vi "WildDrive_v5.0.vi"(6 "Selected_Driver":i32, 8 "Super Turn":bool, 9 "Legal_Drivers":string[](array[string])=["Ethan", "Adam", "Amelia"], 10 "Turn Joystick":dbl, 11 "Speed Joystick":dbl=-0.0) -> (0 "Right Side Power":dbl, 3 "Left Side Power":dbl)   [LabVIEW 2019]
doc: "This VI is designed for use with a butterfly drive, although it can be adapted for use with other differential drive systems. Essentially, this algorithm provides a smooth transition between two different turning modes. At lower speeds the robot will pivot about its center axis while at higher speeds the robot will perform an arc turn. Smooth transitions from deadbands and additional limits on the max pivot turn speed are supported. Toggle \"Turn Behavior\" to steer like car or steer like a traditional FRC robot when driving backwards. Do NOT enter \"Debug Mode\" while the robot is enabled. Do NOT leave \"Synce Driver Profile\" enabled when permenantly deployed to the robot (b/c certain GUI actions are not supported by he RoboRIO). Driver profiles are supported although selection (i.e. via the dashboard) is left to the user."
uses:
  <vilib>/Analysis/1siggen.llb/Ramp Pattern by Samples.vi
  <vilib>/Analysis/NI_AALBase.lvlib
panel:
  in  "Sync Driver Profile":bool
  out "Current_Driver":string
  in  "Feed Forward Coeff":dbl[](array[slide])=[0.05, 0.05, 0.05] min=0.0 max=0.2 scale=0.0..0.2
  in  "Mixing Coefficient":dbl[](array[slide])=[20.0, 20.0, 25.0] min=1.0 max=100.0 scale=1.0..100.0
  in  "Max Pivot Turn (super)":dbl[](array[slide])=[1.0, 1.0, 1.0] min=0.0 max=1.0 scale=0.0..1.0
  in  "Max Pivot Turn (normal)":dbl[](array[slide])=[0.8, 0.8, 0.5] min=0.0 max=1.0 scale=0.0..1.0
  in  "Tune Arc Turn":dbl[](array[slide])=[1.2, 1.2, 0.9] min=0.9 max=2.0 scale=0.9..2.0
  in  "Speed Joystick Deadband":dbl[](array[slide])=[0.05, 0.05, 0.05] min=0.0 max=1.0 scale=0.0..1.0
  in  "Turning Joystick Deadband":dbl[](array[slide])=[0.05, 0.1, 0.2] min=0.0 max=1.0 scale=0.0..1.0
  out "Mixing Function":cluster{"Y":dbl[], "X":dbl[]}(graph)={"Y"=[0.0, 0.010101010101010102, 0.020202020202020204, 0.030303030303030304, 0.04040404040404041, 0.05050505050505051, 0.06060606060606061, 0.07070707070707072, 0.08080808080808081, 0.09090909090909091, 0.10101010101010102, 0.11111111111111112, 0.12121212121212122, 0.13131313131313133, 0.14141414141414144, 0.15151515151515152, 0.16161616161616163, 0.17171717171717174, 0.18181818181818182, 0.19191919191919193, 0.20202020202020204, 0.21212121212121213, 0.22222222222222224, 0.23232323232323235, 0.24242424242424243, 0.25252525252525254, 0.26262626262626265, 0.27272727272727276, 0.2828282828282829, 0.29292929292929293, 0.30303030303030304, 0.31313131313131315, 0.32323232323232326, 0.33333333333333337, 0.3434343434343435, 0.3535353535353536, 0.36363636363636365, 0.37373737373737376, 0.38383838383838387, 0.393939393939394, 0.4040404040404041, 0.4141414141414142, 0.42424242424242425, 0.43434343434343436, 0.4444444444444445, 0.4545454545454546, 0.4646464646464647, 0.4747474747474748, 0.48484848484848486, 0.494949494949495, 0.5050505050505051, 0.5151515151515152, 0.5252525252525253, 0.5353535353535354, 0.5454545454545455, 0.5555555555555556, 0.5656565656565657, 0.5757575757575758, 0.5858585858585859, 0.595959595959596, 0.6060606060606061, 0.6161616161616162, 0.6262626262626263, 0.6363636363636365, 0.6464646464646465, 0.6565656565656566, 0.6666666666666667, 0.6767676767676768, 0.686868686868687, 0.696969696969697, 0.7070707070707072, 0.7171717171717172, 0.7272727272727273, 0.7373737373737375, 0.7474747474747475, 0.7575757575757577, 0.7676767676767677, 0.7777777777777778, 0.787878787878788, 0.797979797979798, 0.8080808080808082, 0.8181818181818182, 0.8282828282828284, 0.8383838383838385, 0.8484848484848485, 0.8585858585858587, 0.8686868686868687, 0.8787878787878789, 0.888888888888889, 0.8989898989898991, 0.9090909090909092, 0.9191919191919192, 0.9292929292929294, 0.9393939393939394, 0.9494949494949496, 0.9595959595959597, 0.9696969696969697, 0.9797979797979799, 0.98989898989899, 1.0], "X"=[1.0, 0.36603234127322715, 0.13532626064379283, 0.05052453015628186, 0.019045702193466962, 0.007247455040202033, 0.002783489278110511, 0.0010787801167675484, 0.00042183410694076207, 0.00016639639425326962, 6.620177984839095e-05, 2.6561398887587357e-05, 1.0745375115522577e-05, 4.382452248980866e-06, 1.8016694372108035e-06, 7.465077591438598e-07, 3.1169901107319554e-07, 1.3113557868070773e-07, 5.5581886768235786e-08, 2.373114697909272e-08, 1.0205242300096137e-08, 4.419721001217318e-09, 1.927446925622597e-09, 8.463234846310681e-10, 3.7411775176233565e-10, 1.6647573596881723e-10, 7.456210476755159e-11, 3.360972414714873e-11, 1.5245699808641053e-11, 6.958609969858144e-12, 3.195570695186819e-12, 1.4763326653758367e-12, 6.86103909791559e-13, 3.2072021853814684e-13, 1.5078403574264123e-13, 7.129180709244532e-14, 3.3895544142624165e-14, 1.6204238353260086e-14, 7.788659967873636e-15, 3.76366378038304e-15, 1.82826621688999e-15, 8.927212895741967e-16, 4.381352486286385e-16, 2.1611505485274178e-16, 1.0713113677174099e-16, 5.336668792886832e-17, 2.6712789155004126e-17, 1.3434882772756658e-17, 6.788690117455716e-18, 3.4462590553247523e-18, 1.7574890123257356e-18, 9.003130684840785e-19, 4.632599227711995e-19, 2.394201316530436e-19, 1.2427288424976475e-19, 6.478095947844572e-20, 3.391170633552417e-20, 1.782623487107148e-20, 9.409232908362009e-21, 4.986671552400837e-21, 2.6534262895136237e-21, 1.4174938853880581e-21, 7.602069865092925e-22, 4.0927762769197154e-22, 2.211867051717034e-22, 1.1998712710421777e-22, 6.53318623500068e-23, 3.570348880574086e-23, 1.958268982155976e-23, 1.0779318073480446e-23, 5.95455071339927e-24, 3.300861649468989e-24, 1.8361511142543956e-24, 1.0248841317144169e-24, 5.739963712987115e-25, 3.2254820658410615e-25, 1.8185053837023498e-25, 1.0286145857915951e-25, 5.837042071494194e-26, 3.3229149745670054e-26, 1.8976510791597504e-26, 1.0870986324891945e-26, 6.246862874883761e-27, 3.6006479544686514e-27, 2.0816633052912476e-27, 1.2070830701485794e-27, 7.020153679465042e-28, 4.094727808938361e-28, 2.3952938868546393e-28, 1.4051883268944269e-28, 8.266830677466088e-29, 4.877074216359946e-29, 2.8852452517622416e-29, 1.711577581520392e-29, 1.0180955963877349e-29, 6.0722055822989395e-30, 3.6312681754960745e-30, 2.1772701780581707e-30, 1.3088709946601708e-30, 7.888609052210118e-31]}
  in  "Debug Mode":bool
  in  "Debug Speed":dbl(slide) min=0.0 max=1.0 scale=0.0..1.0
  in  "Square Speed":bool=TRUE
  in  "Turn Behavior":bool=TRUE
  out "Left Side Power":cluster{"Y":dbl[], "X":dbl[]}(graph)={"Y"=[0.0, 0.010101010101010102, 0.020202020202020204, 0.030303030303030304, 0.04040404040404041, 0.05050505050505051, 0.06060606060606061, 0.07070707070707072, 0.08080808080808081, 0.09090909090909091, 0.10101010101010102, 0.11111111111111112, 0.12121212121212122, 0.13131313131313133, 0.14141414141414144, 0.15151515151515152, 0.16161616161616163, 0.17171717171717174, 0.18181818181818182, 0.19191919191919193, 0.20202020202020204, 0.21212121212121213, 0.22222222222222224, 0.23232323232323235, 0.24242424242424243, 0.25252525252525254, 0.26262626262626265, 0.27272727272727276, 0.2828282828282829, 0.29292929292929293, 0.30303030303030304, 0.31313131313131315, 0.32323232323232326, 0.33333333333333337, 0.3434343434343435, 0.3535353535353536, 0.36363636363636365, 0.37373737373737376, 0.38383838383838387, 0.393939393939394, 0.4040404040404041, 0.4141414141414142, 0.42424242424242425, 0.43434343434343436, 0.4444444444444445, 0.4545454545454546, 0.4646464646464647, 0.4747474747474748, 0.48484848484848486, 0.494949494949495, 0.5050505050505051, 0.5151515151515152, 0.5252525252525253, 0.5353535353535354, 0.5454545454545455, 0.5555555555555556, 0.5656565656565657, 0.5757575757575758, 0.5858585858585859, 0.595959595959596, 0.6060606060606061, 0.6161616161616162, 0.6262626262626263, 0.6363636363636365, 0.6464646464646465, 0.6565656565656566, 0.6666666666666667, 0.6767676767676768, 0.686868686868687, 0.696969696969697, 0.7070707070707072, 0.7171717171717172, 0.7272727272727273, 0.7373737373737375, 0.7474747474747475, 0.7575757575757577, 0.7676767676767677, 0.7777777777777778, 0.787878787878788, 0.797979797979798, 0.8080808080808082, 0.8181818181818182, 0.8282828282828284, 0.8383838383838385, 0.8484848484848485, 0.8585858585858587, 0.8686868686868687, 0.8787878787878789, 0.888888888888889, 0.8989898989898991, 0.9090909090909092, 0.9191919191919192, 0.9292929292929294, 0.9393939393939394, 0.9494949494949496, 0.9595959595959597, 0.9696969696969697, 0.9797979797979799, 0.98989898989899, 1.0], "X"=[0.0]}
  out "Right Side Power":cluster{"Y":dbl[], "X":dbl[]}(graph)={"Y"=[0.0, 0.010101010101010102, 0.020202020202020204, 0.030303030303030304, 0.04040404040404041, 0.05050505050505051, 0.06060606060606061, 0.07070707070707072, 0.08080808080808081, 0.09090909090909091, 0.10101010101010102, 0.11111111111111112, 0.12121212121212122, 0.13131313131313133, 0.14141414141414144, 0.15151515151515152, 0.16161616161616163, 0.17171717171717174, 0.18181818181818182, 0.19191919191919193, 0.20202020202020204, 0.21212121212121213, 0.22222222222222224, 0.23232323232323235, 0.24242424242424243, 0.25252525252525254, 0.26262626262626265, 0.27272727272727276, 0.2828282828282829, 0.29292929292929293, 0.30303030303030304, 0.31313131313131315, 0.32323232323232326, 0.33333333333333337, 0.3434343434343435, 0.3535353535353536, 0.36363636363636365, 0.37373737373737376, 0.38383838383838387, 0.393939393939394, 0.4040404040404041, 0.4141414141414142, 0.42424242424242425, 0.43434343434343436, 0.4444444444444445, 0.4545454545454546, 0.4646464646464647, 0.4747474747474748, 0.48484848484848486, 0.494949494949495, 0.5050505050505051, 0.5151515151515152, 0.5252525252525253, 0.5353535353535354, 0.5454545454545455, 0.5555555555555556, 0.5656565656565657, 0.5757575757575758, 0.5858585858585859, 0.595959595959596, 0.6060606060606061, 0.6161616161616162, 0.6262626262626263, 0.6363636363636365, 0.6464646464646465, 0.6565656565656566, 0.6666666666666667, 0.6767676767676768, 0.686868686868687, 0.696969696969697, 0.7070707070707072, 0.7171717171717172, 0.7272727272727273, 0.7373737373737375, 0.7474747474747475, 0.7575757575757577, 0.7676767676767677, 0.7777777777777778, 0.787878787878788, 0.797979797979798, 0.8080808080808082, 0.8181818181818182, 0.8282828282828284, 0.8383838383838385, 0.8484848484848485, 0.8585858585858587, 0.8686868686868687, 0.8787878787878789, 0.888888888888889, 0.8989898989898991, 0.9090909090909092, 0.9191919191919192, 0.9292929292929294, 0.9393939393939394, 0.9494949494949496, 0.9595959595959597, 0.9696969696969697, 0.9797979797979799, 0.98989898989899, 1.0], "X"=[0.0]}
  out "Speed Joystick Mapping":cluster{"Y":dbl[], "X":dbl[]}(graph)={"Y"=[0.0, 0.010101010101010102, 0.020202020202020204, 0.030303030303030304, 0.04040404040404041, 0.05050505050505051, 0.06060606060606061, 0.07070707070707072, 0.08080808080808081, 0.09090909090909091, 0.10101010101010102, 0.11111111111111112, 0.12121212121212122, 0.13131313131313133, 0.14141414141414144, 0.15151515151515152, 0.16161616161616163, 0.17171717171717174, 0.18181818181818182, 0.19191919191919193, 0.20202020202020204, 0.21212121212121213, 0.22222222222222224, 0.23232323232323235, 0.24242424242424243, 0.25252525252525254, 0.26262626262626265, 0.27272727272727276, 0.2828282828282829, 0.29292929292929293, 0.30303030303030304, 0.31313131313131315, 0.32323232323232326, 0.33333333333333337, 0.3434343434343435, 0.3535353535353536, 0.36363636363636365, 0.37373737373737376, 0.38383838383838387, 0.393939393939394, 0.4040404040404041, 0.4141414141414142, 0.42424242424242425, 0.43434343434343436, 0.4444444444444445, 0.4545454545454546, 0.4646464646464647, 0.4747474747474748, 0.48484848484848486, 0.494949494949495, 0.5050505050505051, 0.5151515151515152, 0.5252525252525253, 0.5353535353535354, 0.5454545454545455, 0.5555555555555556, 0.5656565656565657, 0.5757575757575758, 0.5858585858585859, 0.595959595959596, 0.6060606060606061, 0.6161616161616162, 0.6262626262626263, 0.6363636363636365, 0.6464646464646465, 0.6565656565656566, 0.6666666666666667, 0.6767676767676768, 0.686868686868687, 0.696969696969697, 0.7070707070707072, 0.7171717171717172, 0.7272727272727273, 0.7373737373737375, 0.7474747474747475, 0.7575757575757577, 0.7676767676767677, 0.7777777777777778, 0.787878787878788, 0.797979797979798, 0.8080808080808082, 0.8181818181818182, 0.8282828282828284, 0.8383838383838385, 0.8484848484848485, 0.8585858585858587, 0.8686868686868687, 0.8787878787878789, 0.888888888888889, 0.8989898989898991, 0.9090909090909092, 0.9191919191919192, 0.9292929292929294, 0.9393939393939394, 0.9494949494949496, 0.9595959595959597, 0.9696969696969697, 0.9797979797979799, 0.98989898989899, 1.0], "X"=[0.0]}
  out "Turn Joystick Mapping":cluster{"Y":dbl[], "X":dbl[]}(graph)={"Y"=[0.0, 0.010101010101010102, 0.020202020202020204, 0.030303030303030304, 0.04040404040404041, 0.05050505050505051, 0.06060606060606061, 0.07070707070707072, 0.08080808080808081, 0.09090909090909091, 0.10101010101010102, 0.11111111111111112, 0.12121212121212122, 0.13131313131313133, 0.14141414141414144, 0.15151515151515152, 0.16161616161616163, 0.17171717171717174, 0.18181818181818182, 0.19191919191919193, 0.20202020202020204, 0.21212121212121213, 0.22222222222222224, 0.23232323232323235, 0.24242424242424243, 0.25252525252525254, 0.26262626262626265, 0.27272727272727276, 0.2828282828282829, 0.29292929292929293, 0.30303030303030304, 0.31313131313131315, 0.32323232323232326, 0.33333333333333337, 0.3434343434343435, 0.3535353535353536, 0.36363636363636365, 0.37373737373737376, 0.38383838383838387, 0.393939393939394, 0.4040404040404041, 0.4141414141414142, 0.42424242424242425, 0.43434343434343436, 0.4444444444444445, 0.4545454545454546, 0.4646464646464647, 0.4747474747474748, 0.48484848484848486, 0.494949494949495, 0.5050505050505051, 0.5151515151515152, 0.5252525252525253, 0.5353535353535354, 0.5454545454545455, 0.5555555555555556, 0.5656565656565657, 0.5757575757575758, 0.5858585858585859, 0.595959595959596, 0.6060606060606061, 0.6161616161616162, 0.6262626262626263, 0.6363636363636365, 0.6464646464646465, 0.6565656565656566, 0.6666666666666667, 0.6767676767676768, 0.686868686868687, 0.696969696969697, 0.7070707070707072, 0.7171717171717172, 0.7272727272727273, 0.7373737373737375, 0.7474747474747475, 0.7575757575757577, 0.7676767676767677, 0.7777777777777778, 0.787878787878788, 0.797979797979798, 0.8080808080808082, 0.8181818181818182, 0.8282828282828284, 0.8383838383838385, 0.8484848484848485, 0.8585858585858587, 0.8686868686868687, 0.8787878787878789, 0.888888888888889, 0.8989898989898991, 0.9090909090909092, 0.9191919191919192, 0.9292929292929294, 0.9393939393939394, 0.9494949494949496, 0.9595959595959597, 0.9696969696969697, 0.9797979797979799, 0.98989898989899, 1.0], "X"=[-0.0]}
  # "Driver Inputs"
  # "Tuning Parameters"
  # "Debug"
  # "Drive Outputs"
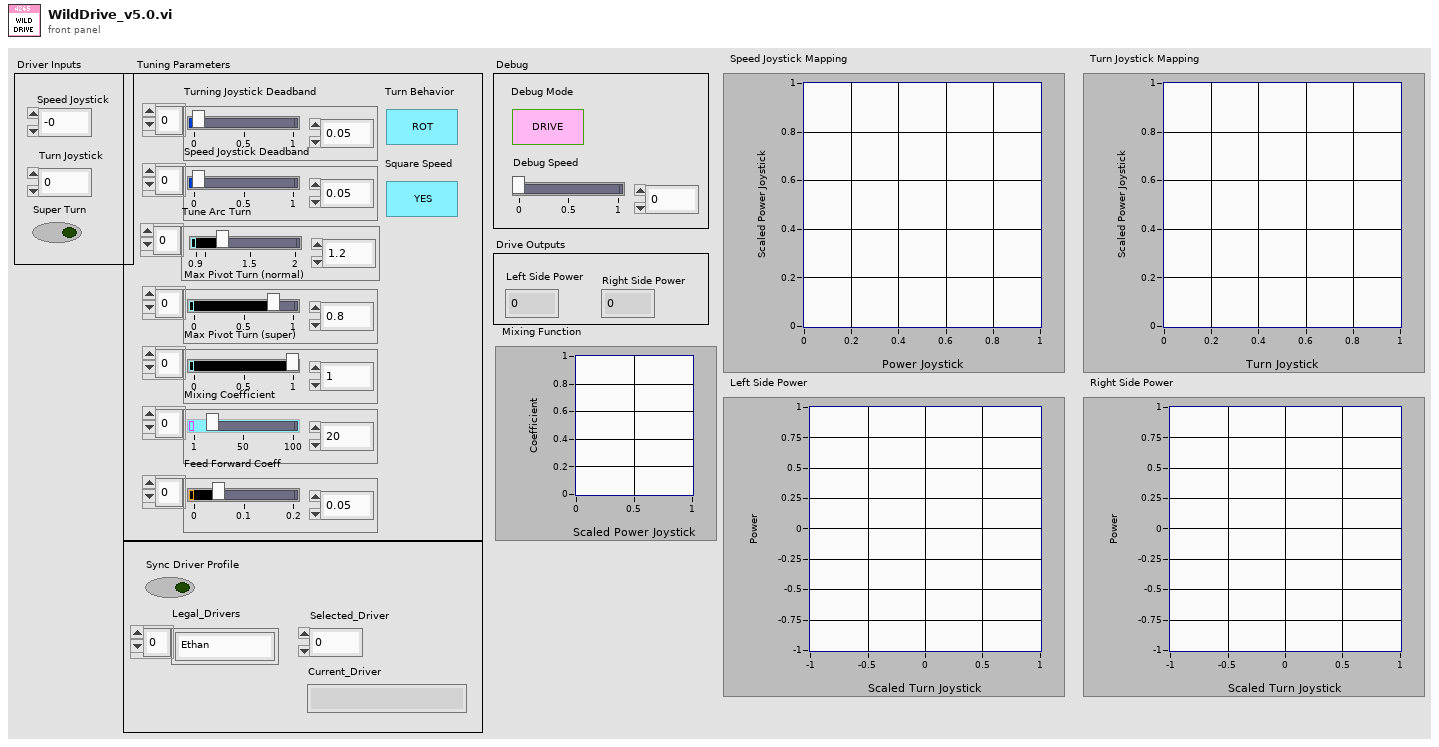
[diagram p1: front panel]
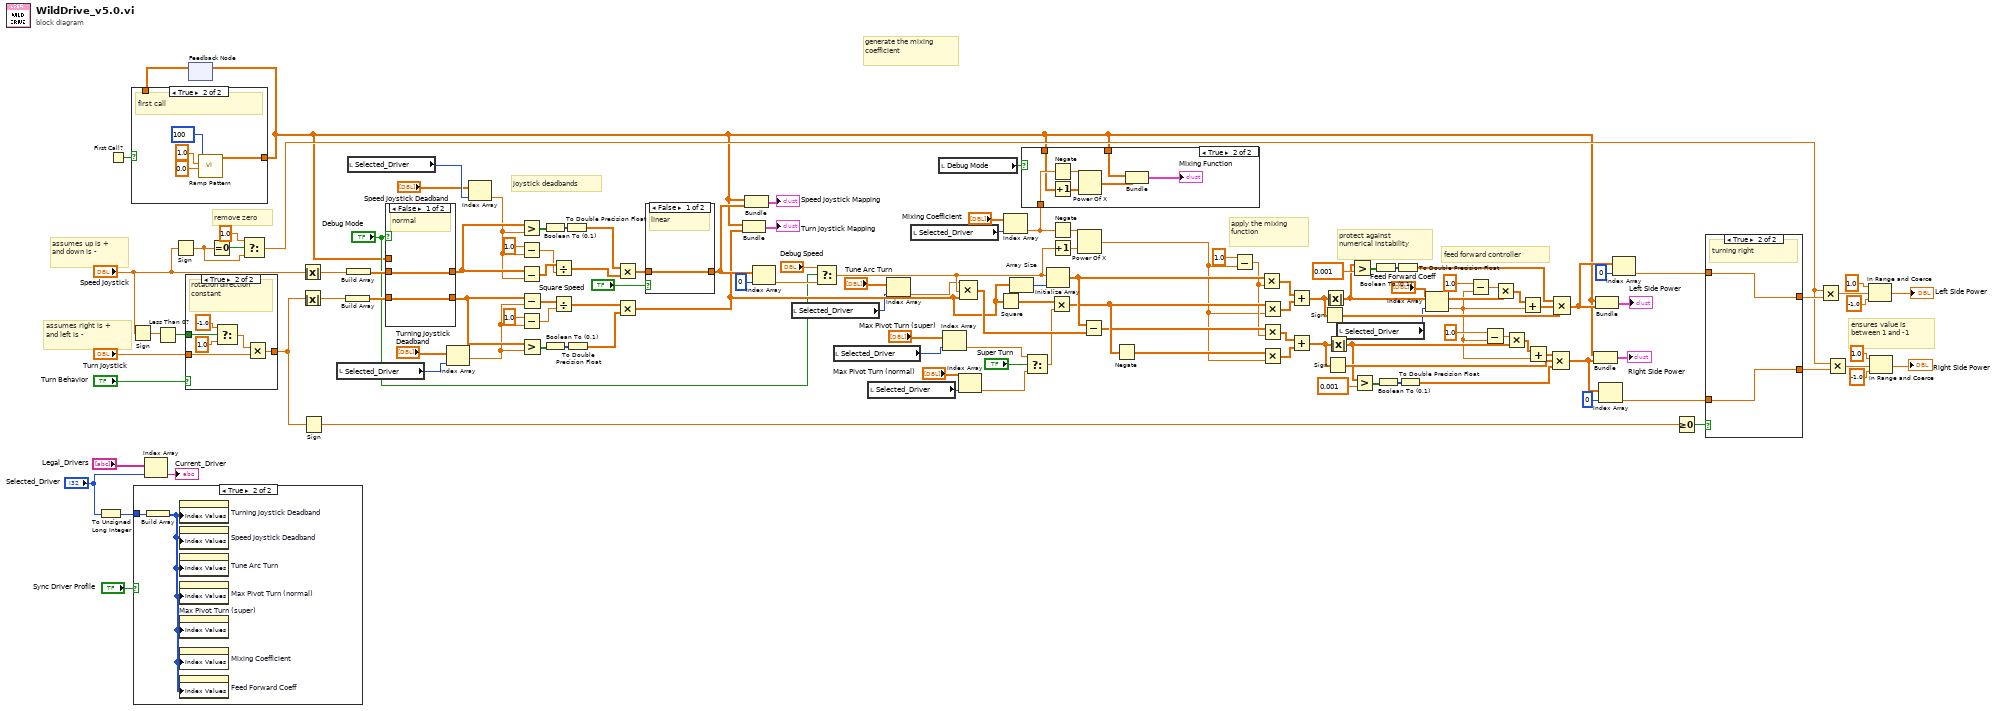
[diagram p0: block diagram]
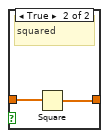
[diagram p8: hidden frame]
diagram:
  # "assumes right is +\nand left is -"
  # "assumes up is +\nand down is -"
  # "apply the mixing\nfunction"
  # "generate the mixing\ncoefficient"
  # "remove zero"
  # "protect against\nnumerical instability"
  # "ensures value is \nbetween 1 and -1"
  # "feed forward controller"
  # "joystick deadbands"
  n1 = To Unsigned Long Integer(number="Selected_Driver") -> (unsigned 32bit integer=w2:u32)
  n2 = First Call?() -> (First Call?: T/F=w52:bool)
  n3 = Sign(1:"Speed Joystick") -> (0:w62:dbl)
  n4 = case shown="True" "Sync Driver Profile" {
    tunnel: w2 -> [_ w133]
    frame False {
    }
    frame True {
      n5 = Build Array(w133) -> (w132:u32[])
      n6 = property on="Turning Joystick Deadband" class="Arr (strict)"("Index Values"=w132) -> ()  [unwired: 2 in, 2 out]
      n7 = property on="Speed Joystick Deadband" class="Arr (strict)"("Index Values"=w132) -> ()  [unwired: 2 in, 2 out]
      n8 = property on="Tune Arc Turn" class="Arr (strict)"("Index Values"=w132) -> ()  [unwired: 2 in, 2 out]
      n9 = property on="Max Pivot Turn (normal)" class="Arr (strict)"("Index Values"=w132) -> ()  [unwired: 2 in, 2 out]
      n10 = property on="Max Pivot Turn (super)" class="Arr (strict)"("Index Values"=w132) -> ()  [unwired: 2 in, 2 out]
      n11 = property on="Mixing Coefficient" class="Arr (strict)"("Index Values"=w132) -> ()  [unwired: 2 in, 2 out]
      n12 = property on="Feed Forward Coeff" class="Arr (strict)"("Index Values"=w132) -> ()  [unwired: 2 in, 2 out]
    }
  }
  n13 = Index Array(array="Legal_Drivers", index="Selected_Driver") -> (element=→"Current_Driver":string)
  n14 = Less Than 0?(x=w62) -> (x < 0?=w63:bool)
  n15 = Sign(1:"Speed Joystick") -> (0:w55:dbl)
  n16 = case shown="True" "Turn Behavior" {
    tunnel: w63 -> [_ w139]
    tunnel: [w134 w136] -> w58
    tunnel: "Turn Joystick" -> [w134 w135]
    frame False {
      # "like a car"
    }
    frame True {
      # "rotation direction constant"
      n17 = Select(t=-1.0, s=w139, f=1.0) -> (s? t:f=w140:dbl)
      n18 = Multiply(x=w140, y=w135) -> (x*y=w136:dbl)
    }
  }
  n19 = feedback #1() -> (w51:dbl[])  [unwired: 1 in]
  n20 = case shown="True" w52 {
    tunnel: [w141 w142] -> w28
    tunnel: w51 -> [w141 _]
    frame False {
      # "subsequent calls"
    }
    frame True {
      # "first call"
      n21 = call-poly <vilib>:"Ramp Pattern.vi"("start"=0.0, "end"=1.0, "samples"=100) -> ("Ramp Pattern"=w142:dbl[])  [unwired: 7 in, 1 out]
    }
  }
  n22 = feedback-in #1(w28) -> ()
  n23 = Equal To 0?(x=w55) -> (x = 0?=w57:bool)
  n24 = Select(t=1.0, s=w57, f=w55) -> (s? t:f=w54:dbl)
  n25 = Absolute Value(x="Speed Joystick") -> (abs(x)=w128:dbl)
  n26 = Absolute Value(x=w58) -> (abs(x)=w131:dbl)
  n27 = Sign(1:w58) -> (0:w66:dbl)
  n28 = local read "Selected_Driver"() -> (w24:i32)
  n29 = Build Array(w131) -> (w129:dbl[])
  n30 = Build Array(w128) -> (w130:dbl[])
  n31 = local read "Selected_Driver"() -> (w23:i32)
  n32 = case shown="False" "Debug Mode" {
    tunnel: w28 -> [_ w148]
    tunnel: [w147 w148] -> w119
    tunnel: [w146 w148] -> w111
    tunnel: w130 -> [w147 _]
    tunnel: w129 -> [w146 _]
    frame False {
      # "normal"
    }
    frame True {
      # "debug"
    }
  }
  n33 = Index Array(array="Turning Joystick Deadband", index=w24) -> (element=w25:dbl)
  n34 = Index Array(array="Speed Joystick Deadband", index=w23) -> (element=w22:dbl)
  n35 = Greater?(x=w119, y=w22) -> (0:w125:bool[])
  n36 = Subtract(x=1.0, y=w22) -> (x-y=w116:dbl)
  n37 = Subtract(x=w119, y=w22) -> (x-y=w118:dbl[])
  n38 = Subtract(x=1.0, y=w25) -> (x-y=w112:dbl)
  n39 = Subtract(x=w111, y=w25) -> (x-y=w114:dbl[])
  n40 = Greater?(x=w111, y=w25) -> (0:w123:bool[])
  n41 = Boolean To (0,1)(Boolean=w125) -> (0, 1=w124:i16[])
  n42 = Boolean To (0,1)(Boolean=w123) -> (0, 1=w122:i16[])
  n43 = Divide(x=w118, y=w116) -> (x/y=w115:dbl[])
  n44 = Divide(x=w114, y=w112) -> (x/y=w110:dbl[])
  n45 = To Double Precision Float(number=w124) -> (double precision float=w121:dbl[])
  n46 = To Double Precision Float(number=w122) -> (double precision float=w109:dbl[])
  n47 = Multiply(x=w121, y=w115) -> (x*y=w120:dbl[])
  n48 = Multiply(x=w110, y=w109) -> (x*y=w47:dbl[])
  n49 = case shown="False" "Square Speed" {
    tunnel: w120 -> [w149 w151]
    tunnel: [w149 w150] -> w102
    frame False {
      # "linear"
    }
    frame True {
      # "squared"
      n50 = Square(x=w151) -> (x^2=w150:dbl[])
    }
  }
  n51 = Bundle("Ramp Pattern"=w28, w47) -> (→"Turn Joystick Mapping":cluster{"Ramp Pattern":dbl[], dbl[]})  [unwired: 1 in]
  n52 = Bundle("Ramp Pattern"=w28, w102) -> (→"Speed Joystick Mapping":cluster{"Ramp Pattern":dbl[], dbl[]})  [unwired: 1 in]
  n53 = Index Array(array=w102, index=0) -> (element=w104:dbl)
  n54 = local read "Selected_Driver"() -> (w19:i32)
  n55 = Select(t="Debug Speed", s="Debug Mode", f=w104) -> (s? t:f=w32:dbl)
  n56 = local read "Selected_Driver"() -> (w13:i32)
  n57 = local read "Selected_Driver"() -> (w17:i32)
  n58 = Index Array(array="Tune Arc Turn", index=w19) -> (element=w18:dbl)
  n59 = local read "Selected_Driver"() -> (w9:i32)
  n60 = local read "Debug Mode"() -> (w27:bool)
  n61 = Index Array(array="Max Pivot Turn (super)", index=w13) -> (element=w12:dbl)
  n62 = Index Array(array="Max Pivot Turn (normal)", index=w17) -> (element=w15:dbl)
  n63 = Compound Arithmetic op=MULTIPLY(w18, w32, w47) -> (w105:dbl[])
  n64 = Square(x=w47) -> (x^2=w53:dbl[])
  n65 = Index Array(array="Mixing Coefficient", index=w9) -> (element=w11:dbl)
  n66 = Array Size(array=w47) -> (size(s)=w108:i32)
  n67 = case shown="True" w27 {
    tunnel: w11 -> [_ w156]
    tunnel: w28 -> [_ w154]
    tunnel: w28 -> [_ w152]
    frame False {
    }
    frame True {
      n68 = Negate(x=w156) -> (-x=w158:dbl)
      n69 = Increment(x=w154) -> (x+1=w157:dbl[])
      n70 = Power Of X(1:w157, 2:w158) -> (0:w153:dbl[])
      n71 = Bundle("Ramp Pattern"=w152, w153) -> (→"Mixing Function":cluster{"Ramp Pattern":dbl[], dbl[]})  [unwired: 1 in]
    }
  }
  n72 = Select(t=w12, s="Super Turn", f=w15) -> (s? t:f=w50:dbl)
  n73 = Initialize Array(w32, w108) -> (w44:dbl[])
  n74 = Multiply(x=w53, y=w50) -> (x*y=w43:dbl[])
  n75 = Negate(x=w11) -> (-x=w31:dbl)
  n76 = Increment(x=w32) -> (x+1=w30:dbl)
  n77 = Power Of X(1:w30, 2:w31) -> (0:w29:dbl)
  n78 = Subtract(x=w44, y=w105) -> (x-y=w37:dbl[])
  n79 = Negate(x=w43) -> (-x=w36:dbl[])
  n80 = Subtract(x=1.0, y=w29) -> (x-y=w33:dbl)
  n81 = Multiply(x=w44, y=w33) -> (x*y=w42:dbl[])
  n82 = Multiply(x=w43, y=w29) -> (x*y=w41:dbl[])
  n83 = Multiply(x=w37, y=w33) -> (x*y=w39:dbl[])
  n84 = Multiply(x=w36, y=w29) -> (x*y=w38:dbl[])
  n85 = Add(x=w42, y=w41) -> (x+y=w40:dbl[])
  n86 = Add(x=w39, y=w38) -> (x+y=w35:dbl[])
  n87 = Sign(1:w40) -> (0:w98:dbl[])
  n88 = Absolute Value(x=w40) -> (abs(x)=w64:dbl[])
  n89 = Sign(1:w35) -> (0:w93:dbl[])
  n90 = Absolute Value(x=w35) -> (abs(x)=w65:dbl[])
  n91 = local read "Selected_Driver"() -> (w6:i32)
  n92 = Greater?(x=w64, y=0.001) -> (0:w88:bool[])
  n93 = Greater?(x=w65, y=0.001) -> (0:w92:bool[])
  n94 = Boolean To (0,1)(Boolean=w88) -> (0, 1=w87:i16[])
  n95 = Boolean To (0,1)(Boolean=w92) -> (0, 1=w91:i16[])
  n96 = To Double Precision Float(number=w87) -> (double precision float=w85:dbl[])
  n97 = To Double Precision Float(number=w91) -> (double precision float=w89:dbl[])
  n98 = Index Array(array="Feed Forward Coeff", index=w6) -> (element=w8:dbl)
  n99 = Subtract(x=1.0, y=w8) -> (x-y=w100:dbl)
  n100 = Subtract(x=1.0, y=w8) -> (x-y=w96:dbl)
  n101 = Multiply(x=w100, y=w64) -> (x*y=w99:dbl[])
  n102 = Multiply(x=w96, y=w65) -> (x*y=w95:dbl[])
  n103 = Add(x=w99, y=w8) -> (x+y=w84:dbl[])
  n104 = Add(x=w95, y=w8) -> (x+y=w94:dbl[])
  n105 = Compound Arithmetic op=MULTIPLY(w94, w93, w89) -> (w82:dbl[])
  n106 = Compound Arithmetic op=MULTIPLY(w85, w84, w98) -> (w80:dbl[])
  n107 = Bundle("Ramp Pattern"=w28, w82) -> (→"Right Side Power":cluster{"Ramp Pattern":dbl[], dbl[]})  [unwired: 1 in]
  n108 = Bundle("Ramp Pattern"=w28, w80) -> (→"Left Side Power":cluster{"Ramp Pattern":dbl[], dbl[]})  [unwired: 1 in]
  n109 = Index Array(array=w82, index=0) -> (element=w69:dbl)
  n110 = Index Array(array=w80, index=0) -> (element=w71:dbl)
  n111 = Greater Or Equal To 0?(x=w66) -> (x >= 0?=w67:bool)
  n112 = case shown="True" w67 {
    tunnel: w71 -> [w160 w162]
    tunnel: [w159 w162] -> w70
    tunnel: w69 -> [w159 w161]
    tunnel: [w160 w161] -> w68
    frame False {
      # "turning left"
    }
    frame True {
      # "turning right"
    }
  }
  n113 = Multiply(x=w54, y=w70) -> (x*y=w72:dbl)
  n114 = Multiply(x=w54, y=w68) -> (x*y=w73:dbl)
  n115 = In Range and Coerce(upper limit=1.0, x=w72, lower limit=-1.0) -> (coerced(x)=→"Left Side Power":dbl)  [unwired: 1 out]
  n116 = In Range and Coerce(upper limit=1.0, x=w73, lower limit=-1.0) -> (coerced(x)=→"Right Side Power":dbl)  [unwired: 1 out]
